vi "RichToFlatni_measurementlink_pinmap_v1_ResourceAccessInformation.vi"(5 "OutputClusterType":T1, 11 "InputCluster":T3) -> (3 "OutputCluster":T1)   [LabVIEW 2021, in "ni.measurementlink.pinmap.v1.api.lvlib"]
uses:
  ni_measurementlink_pinmap_v1_ResourceAccessInformation.ctl
  ni_measurementlink_pinmap_v1_ChannelMapping.ctl
  ni_measurementlink_pinmap_v1_ResourceAccessInformation_Flat.ctl
  ni_measurementlink_pinmap_v1_ChannelMapping_Flat.ctl
  ni.measurementlink.pinmap.v1.api.lvlib
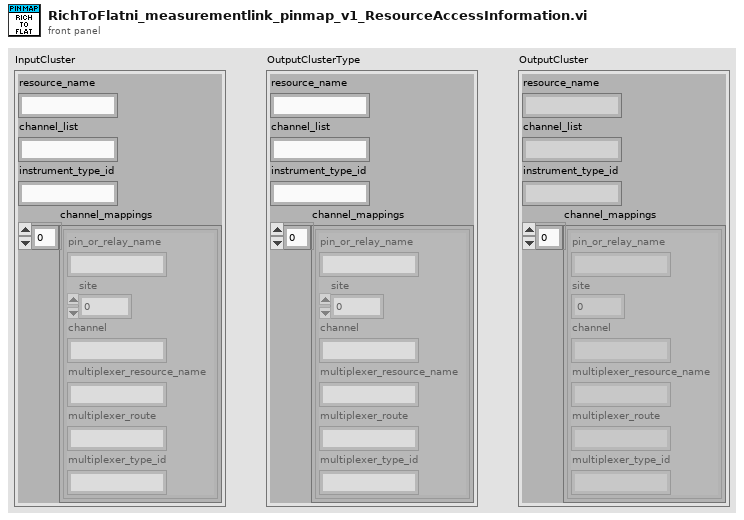
[diagram p1: front panel]
types:
  T1 = typedef "ni.measurementlink.pinmap.v1.api.lvlib/ni_measurementlink_pinmap_v1_ResourceAccessInformation_Flat.ctl" = cluster{"resource_name":string, "channel_list":string, "instrument_type_id":string, "channel_mappings":T2[]}
  T2 = typedef "ni.measurementlink.pinmap.v1.api.lvlib/ni_measurementlink_pinmap_v1_ChannelMapping_Flat.ctl" = cluster{"pin_or_relay_name":string, "site":i32, "channel":string, "multiplexer_resource_name":string, "multiplexer_route":string, "multiplexer_type_id":string}
  T3 = typedef "ni.measurementlink.pinmap.v1.api.lvlib/ni_measurementlink_pinmap_v1_ResourceAccessInformation.ctl" = cluster{"resource_name":string, "channel_list":string, "instrument_type_id":string, "channel_mappings":T4[]}
  T4 = typedef "ni.measurementlink.pinmap.v1.api.lvlib/ni_measurementlink_pinmap_v1_ChannelMapping.ctl" = cluster{"pin_or_relay_name":string, "site":i32, "channel":string, "multiplexer_resource_name":string, "multiplexer_route":string, "multiplexer_type_id":string}
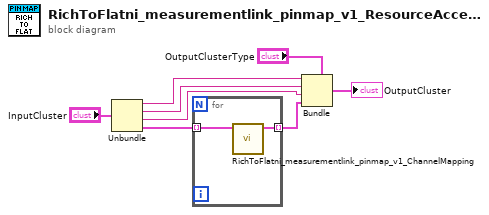
[diagram p0: block diagram]
diagram:
  n1 = Unbundle "Unbundle"("InputCluster") -> ("resource_name"=w5:string, "channel_list"=w4:string, "instrument_type_id"=w3:string, "channel_mappings"=w2:T4[])
  n2 = for {
    tunnel: w2 -> [w10] mode=indexing
    tunnel: [w9] -> w1 mode=indexing
    n3 = call "RichToFlatni_measurementlink_pinmap_v1_ChannelMapping.vi"("InputCluster"=w10) -> ("OutputCluster"=w9:T2)  [unwired: 10 in]
  }
  n4 = Bundle "Bundle"(cluster="OutputClusterType", "resource_name"=w5, "channel_list"=w4, "instrument_type_id"=w3, "channel_mappings"=w1) -> (→"OutputCluster":T1)
